vi "Plasma etching vacuum chamber automatization.vi"() -> ()   [LabVIEW 2019]
uses:
  <vilib>/MakerHub/LINX/Private/Type Defs/User Platform.ctl
  <vilib>/MakerHub/LINX/Public/Peripherals/Digital/Digital Read N Chans.vi
  <vilib>/MakerHub/LINX/Public/Peripherals/Digital/Digital Write N Chans.vi
  <vilib>/MakerHub/LINX/Public/Peripherals/Analog/Analog Read N Chans.vi
  <vilib>/MakerHub/LINX/Private/Local IO/LinxDigitalRead.vi
  <vilib>/MakerHub/LINX/Public/Utilities/Check Channel.vi
  <vilib>/MakerHub/LINX/Private/Local IO/LinxDigitalWrite.vi
  <vilib>/MakerHub/LINX/Private/Local IO/LinxAnalogRead.vi
  <vilib>/MakerHub/LINX/Private/Utilties/Generate Error.vi
  <vilib>/MakerHub/LINX/LMH-LINX.lvlib
panel:
  out "DIFFUSION PUMP HEATER VAR":bool
  in  "Tab Control":T1(tab)
  out "Back Air Admit":bool
  out "Chamber Valve":bool
  out "DIFF Valve":bool
  out "DIFFUSION PUMP Heater":bool
  out "Diafragma":bool
  out "Woter Exist":bool
  in  "Cold Woter Chamber":bool
  in  "Hot Woter  Chamber":bool
  out "Chamber Air Admit":bool
  out "Diff Pump Hot":bool
  out "Mechanic Pump":bool
  in  "Chamber Air Admit 2":bool
  out "Down Space Low Vacuum":dbl(knob) scale=0.0..1.0 scale format="%#_2g"
  in  "Chamber Open":bool
  in  "Chamber Close":bool
  out "Self Pumping":bool
  in  "Auto Start":bool
  in  "END Process":bool
  in  "STOP":bool
  out "Process Succesful ENDED":bool
  out "Vacuum Good":bool
  out "Chamber Low Vacuum":dbl(knob) scale=0.0..1.0 scale format="%#_2g"
  in  "Manual/Auto":bool
  out "Vacuum Measure":dbl(graph)
  out "High Vacuum Pascal":dbl format="%#_2e"
  in  "Serial Port":refnum<visa-resource-name>="COM12"
  in  "Diafragma Manual":bool
  in  "air Admit Manual":bool
  in  "Diff Pump Manual":bool
  in  "Chamber air Admit Manual":bool
  in  "DIFF VALVE Manual":bool
  in  "Mechanical Pump Manual":bool
  in  "CHAMBER VALVE Manual":bool
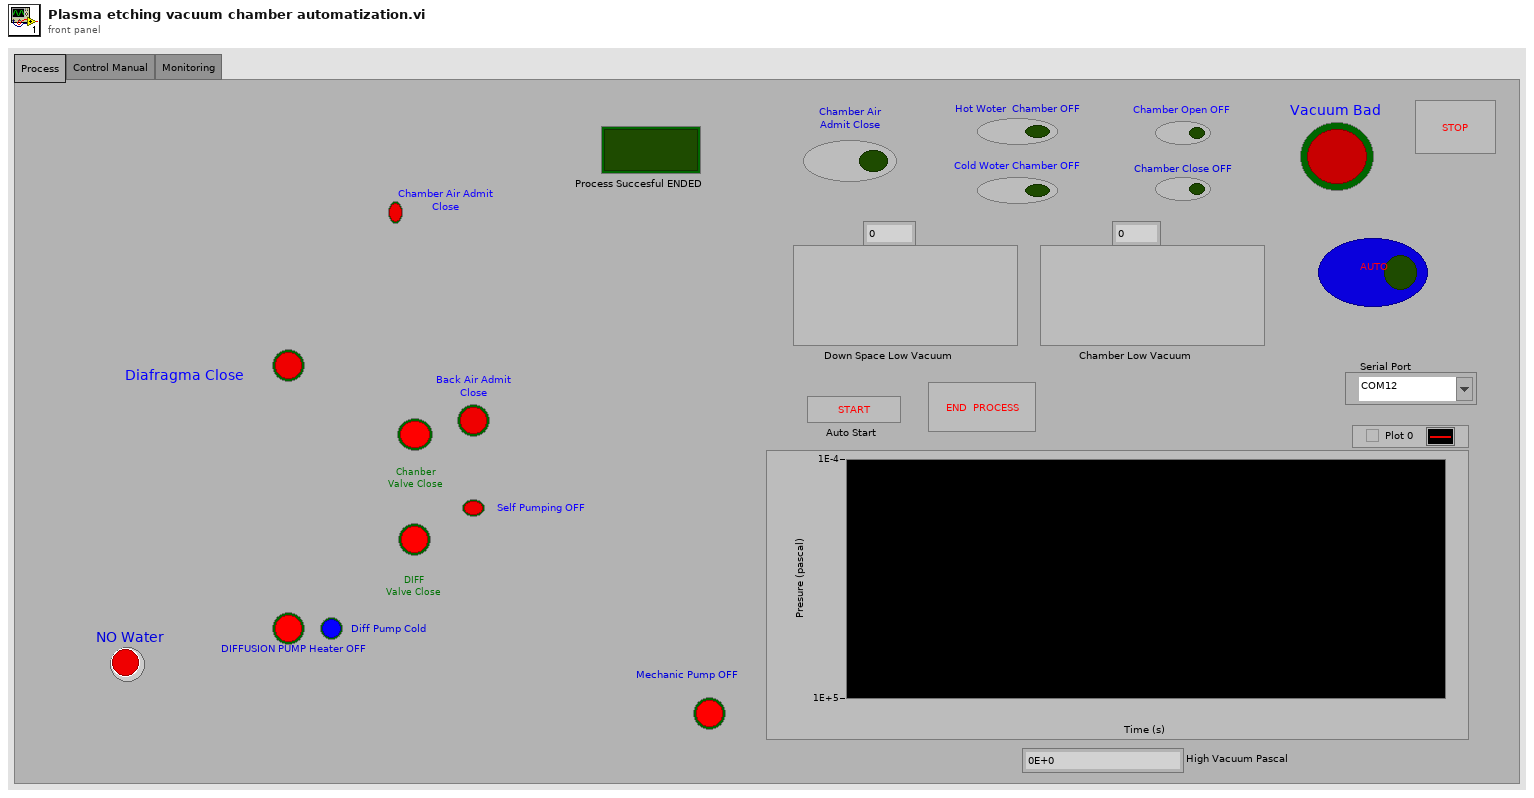
[diagram p1: front panel]
types:
  T1 = enum32{"Process", "Control Manual", "Monitoring"}
  T2 = typedef "LMH-LINX.lvlib/User Platform.ctl" = enum16{"Default", "Remote", "Local"}
  T3 = typedef "LMH-LINX.lvlib/LINX Ref.ctl" = cluster{"IO":T4, "Interface":T5, "LINX Device Config":T6}
  T4 = typedef "LMH-LINX.lvlib/Platform.ctl" = enum16{"Remote", "Local"}
  T5 = typedef "LMH-LINX.lvlib/Interface.ctl" = enum16{"Serial", "TCP"}
  T6 = typedef "LMH-LINX.lvlib/Device.lvlib/LINX Device Config.ctl" = cluster{"Interface":T5, "COM Port":refnum<visa-resource-name>, "TCP Configuration":T7, "Device Family":u8, "Device ID":u8, "Device Name":string, "TCP Ref":refnum<k5>, "Channels":T8}
  T7 = typedef "LMH-LINX.lvlib/Device.lvlib/TCP Config.ctl" = cluster{"IP Address":string, "Port":u16}
  T8 = typedef "LMH-LINX.lvlib/Channels.ctl" = cluster{"DI":u8[], "DO":u8[], "AI":u8[], "AO":u8[], "PWM":u8[], "QE":u8[], "UART":u8[], "I2C 2":u8[], "SPI":u8[], "CAN":u8[], "Servo":u8[], "AI Ref (V)":dbl, "AI Resolution (Bits)":u8, "AO Ref (V)":dbl, "AO Resolution (Bits)":u8}
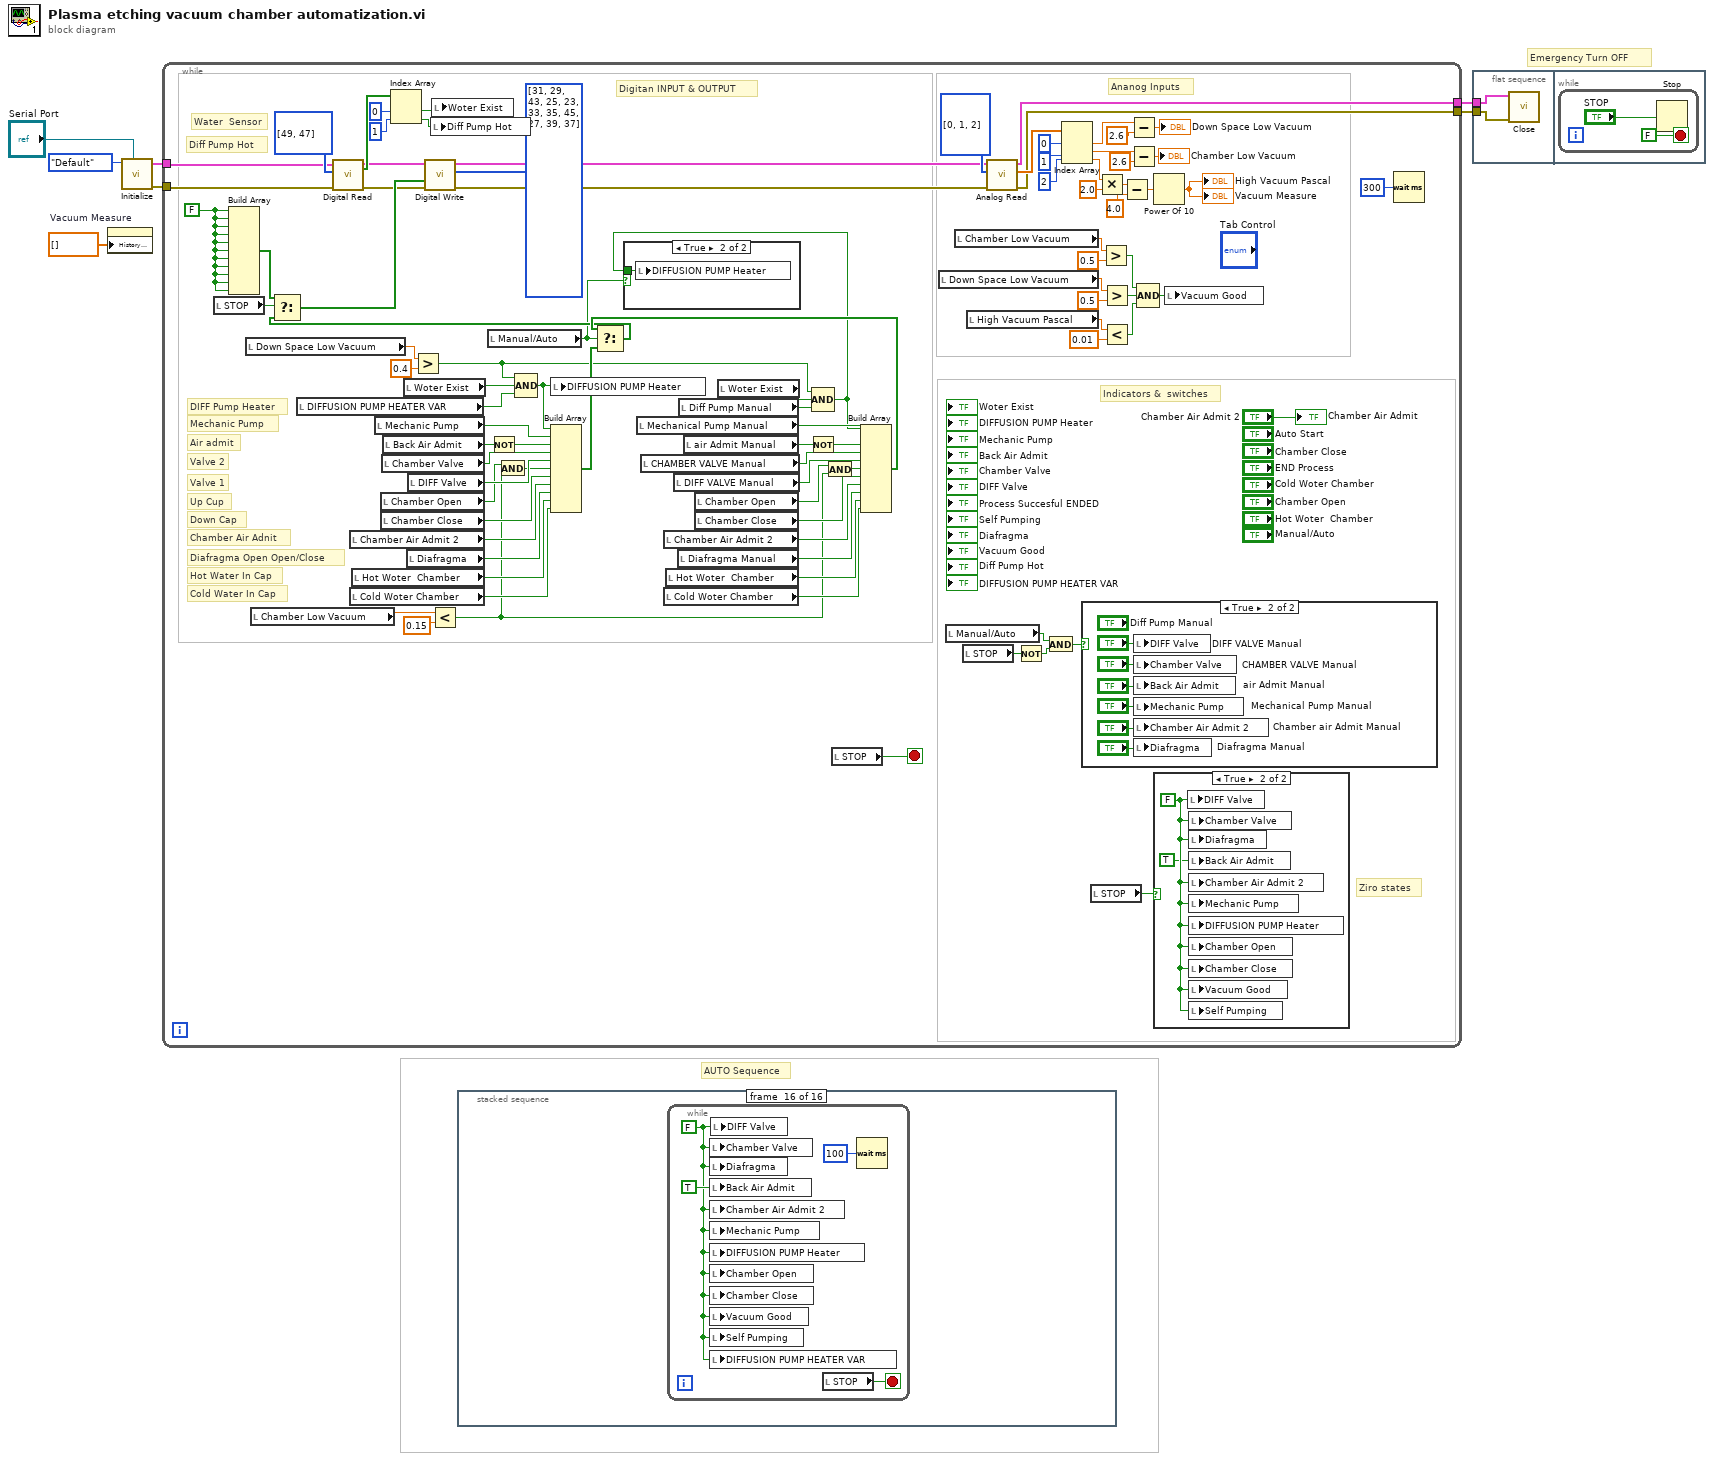
[diagram p0: block diagram]
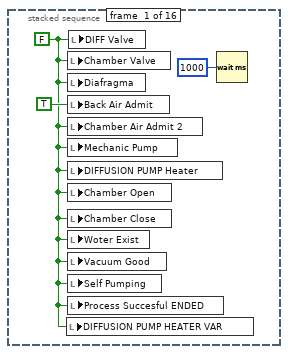
[diagram p2: hidden frame]
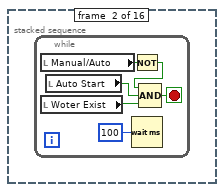
[diagram p3: hidden frame]
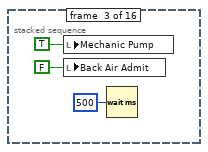
[diagram p4: hidden frame]
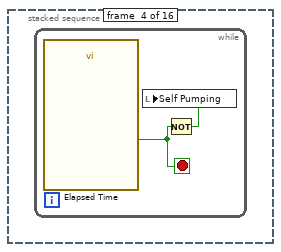
[diagram p5: hidden frame]
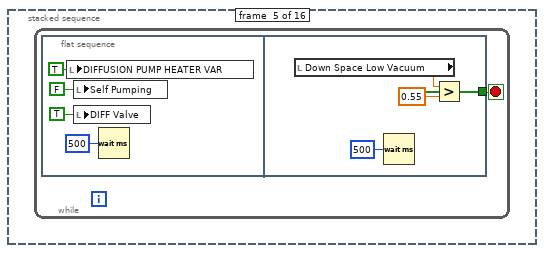
[diagram p6: hidden frame]
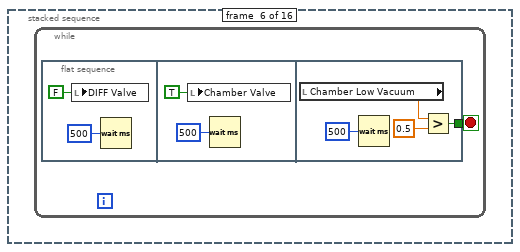
[diagram p7: hidden frame]
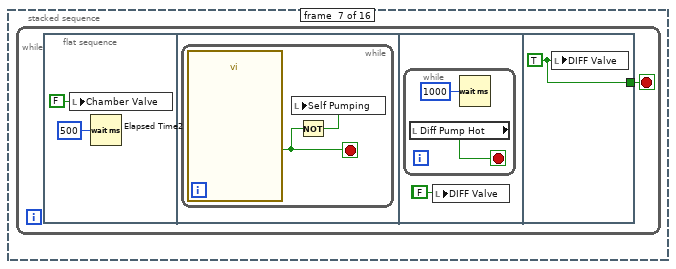
[diagram p8: hidden frame]
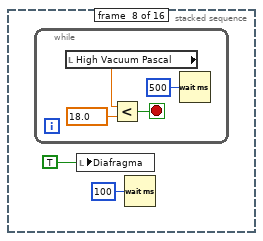
[diagram p9: hidden frame]
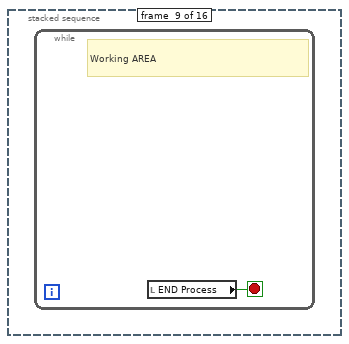
[diagram p10: hidden frame]
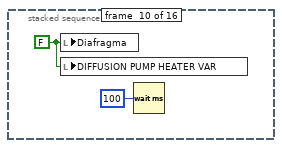
[diagram p11: hidden frame]
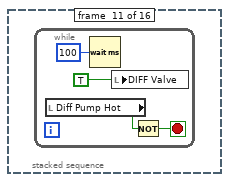
[diagram p12: hidden frame]
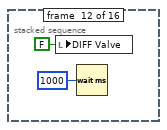
[diagram p13: hidden frame]
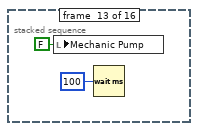
[diagram p14: hidden frame]
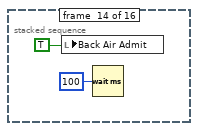
[diagram p15: hidden frame]
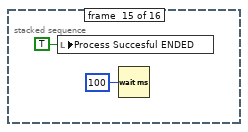
[diagram p16: hidden frame]
diagram:
  # "Emergency Turn OFF"
  # "AUTO Sequence"
  n1 = property on="Vacuum Measure" class="WFChart (strict)"("History Data"=dbl[] []) -> ()  [unwired: 2 in, 2 out]
  n2 = call <vilib>:"Initialize.vi"("Serial Port"="Serial Port", "IO"=User_Platform."Default" ("Platform")) -> ("Error Out"=w4:errorcluster, "LINX Resource"=w5:T3)  [unwired: 7 in, 1 out]
  n3 = while {
    tunnel: w5 -> [w52]
    tunnel: w4 -> [w51]
    tunnel: [w11] -> w3
    tunnel: [w10] -> w2
    stop <- w9 stop-if-true
    w58 = FALSE ("element")
    # "Ziro states"
    # "Indicators &  switches"
    # "Ananog Inputs"
    # "Diff Pump Hot"
    # "Cold Water In Cap"
    # "Hot Water In Cap"
    # "Diafragma Open Open/Close"
    # "Chamber Air Adnit"
    # "Down Cap"
    # "Up Cup"
    # "DIFF Pump Heater"
    # "Mechanic Pump"
    # "Air admit"
    # "Valve 2"
    # "Valve 1"
    # "Water  Sensor"
    # "Digitan INPUT & OUTPUT"
    n4 = local read "STOP"() -> (w54:bool)
    n5 = Build Array(w58, w58, w58, w58, w58, w58, w58, w58, w58, w58, w58) -> (w57:bool[])
    n6 = local read "Down Space Low Vacuum"() -> (w78:dbl)
    n7 = local read "Chamber Low Vacuum"() -> (w81:dbl)
    n8 = local read "DIFFUSION PUMP HEATER VAR"() -> (w59:bool)
    n9 = call-poly <vilib>:"Digital Read.vi"("Error In"=w51, "DI Channels"=u8[] [49, 47], "LINX Resource"=w52) -> ("Error Out"=w21:errorcluster, "Values"=w100:bool[], "LINX Resource"=w22:T3)  [unwired: 6 in]
    n10 = local read "Chamber Air Admit 2"() -> (w91:bool)
    n11 = local read "Cold Woter Chamber"() -> (w86:bool)
    n12 = local read "Hot Woter  Chamber"() -> (w87:bool)
    n13 = local read "Mechanic Pump"() -> (w98:bool)
    n14 = local read "Chamber Open"() -> (w82:bool)
    n15 = local read "Chamber Close"() -> (w92:bool)
    n16 = local read "Chamber Valve"() -> (w96:bool)
    n17 = local read "Back Air Admit"() -> (w84:bool)
    n18 = Index Array(array=w100, index #1=0 ("index"), index #2=1 ("index")) -> (element #1=w101:bool, element #2=w88:bool)
    n19 = local read "Woter Exist"() -> (w79:bool)
    n20 = local read "Diafragma"() -> (w90:bool)
    n21 = local read "DIFF Valve"() -> (w97:bool)
    n22 = Greater?(x=w78, y=0.4) -> (0:w63:bool)
    n23 = Less?(x=w81, y=0.15) -> (x < y?=w62:bool)
    n24 = local write "Diff Pump Hot"(w88) -> ()
    n25 = local write "Woter Exist"(w101) -> ()
    n26 = local read "Manual/Auto"() -> (w48:bool)
    n27 = Not(x=w84) -> (.not. x?=w85:bool)
    n28 = And(x=w82, y=w62) -> (x .and. y?=w83:bool)
    n29 = Compound Arithmetic op=AND(w63, w79, w59) -> (w60:bool)
    n30 = local write "DIFFUSION PUMP Heater"(w60) -> ()
    n31 = Build Array(w60, w98, w85, w96, w97, w83, w92, w91, w90, w87, w86) -> (w64:bool[])
    n32 = local read "Mechanical Pump Manual"() -> (w67:bool)
    n33 = local read "CHAMBER VALVE Manual"() -> (w66:bool)
    n34 = local read "Chamber Air Admit 2"() -> (w72:bool)
    n35 = local read "Cold Woter Chamber"() -> (w75:bool)
    n36 = local read "Hot Woter  Chamber"() -> (w74:bool)
    n37 = local read "DIFF VALVE Manual"() -> (w65:bool)
    n38 = local read "Diafragma Manual"() -> (w73:bool)
    n39 = local read "Diff Pump Manual"() -> (w49:bool)
    n40 = local read "air Admit Manual"() -> (w70:bool)
    n41 = local read "Chamber Open"() -> (w50:bool)
    n42 = local read "Chamber Close"() -> (w71:bool)
    n43 = local read "Woter Exist"() -> (w68:bool)
    n44 = Not(x=w70) -> (.not. x?=w69:bool)
    n45 = Compound Arithmetic op=AND(w63, w68, w49) -> (w53:bool)
    n46 = case shown="True" w48 {
      tunnel: w53 -> [_ w110]
      frame False {
      }
      frame True {
        n47 = local write "DIFFUSION PUMP Heater"(w110) -> ()
      }
    }
    n48 = And(x=w50, y=w62) -> (x .and. y?=w61:bool)
    n49 = local read "STOP"() -> (w9:bool)
    n50 = Build Array(w53, w67, w69, w66, w65, w61, w71, w72, w73, w74, w75) -> (w76:bool[])
    n51 = Select(t=w76, s=w48, f=w64) -> (s? t:f=w55:bool[])
    n52 = Select(t=w57, s=w54, f=w55) -> (s? t:f=w56:bool[])
    n53 = call-poly <vilib>:"Digital Write.vi"("Error In"=w21, "Values"=w56, "DO Channels"=u8[] [31, 29, 43, 25, 23, 33, 35, 45, 27, 39, 37], "LINX Resource"=w22) -> ("Error Out"=w19:errorcluster, "LINX Resource"=w20:T3)  [unwired: 6 in]
    n54 = local read "Down Space Low Vacuum"() -> (w33:dbl)
    n55 = local read "Manual/Auto"() -> (w14:bool)
    n56 = local read "Chamber Low Vacuum"() -> (w36:dbl)
    n57 = local read "STOP"() -> (w13:bool)
    n58 = local read "High Vacuum Pascal"() -> (w32:dbl)
    n59 = call-poly <vilib>:"Analog Read.vi"("Error In"=w19, "AI Channel(s)"=u8[] [0, 1, 2], "LINX Resource"=w20) -> ("Error Out"=w10:errorcluster, "Voltages"=w27:dbl[], "LINX Resource"=w11:T3)  [unwired: 5 in, 1 out]
    n60 = Not(x=w13) -> (.not. x?=w12:bool)
    n61 = And(x=w14, y=w12) -> (x .and. y?=w15:bool)
    n62 = Index Array(array=w27, index #1=0 ("index"), index #2=1 ("index"), index #3=2 ("index")) -> (element #1=w28:dbl, element #2=w41:dbl, element #3=w18:dbl)
    n63 = case shown="True" w15 {
      frame False {
      }
      frame True {
        n64 = local write "DIFF Valve"("DIFF VALVE Manual") -> ()
        n65 = local write "Chamber Valve"("CHAMBER VALVE Manual") -> ()
        n66 = local write "Back Air Admit"("air Admit Manual") -> ()
        n67 = local write "Mechanic Pump"("Mechanical Pump Manual") -> ()
        n68 = local write "Chamber Air Admit 2"("Chamber air Admit Manual") -> ()
        n69 = local write "Diafragma"("Diafragma Manual") -> ()
      }
    }
    n70 = local read "STOP"() -> (w8:bool)
    n71 = Multiply(x=w18, y=2.0 ("x")) -> (x*y=w47:dbl)
    n72 = Greater?(x=w36, y=0.5) -> (0:w37:bool)
    n73 = Greater?(x=w33, y=0.5) -> (0:w38:bool)
    n74 = Less?(x=w32, y=0.01) -> (x < y?=w39:bool)
    n75 = Subtract(x=w47, y=4.0) -> (x-y=w45:dbl)
    n76 = Subtract(x=w28, y=2.6) -> (x-y=→"Down Space Low Vacuum":dbl)
    n77 = Subtract(x=w41, y=2.6) -> (x-y=→"Chamber Low Vacuum":dbl)
    n78 = Compound Arithmetic op=AND(w37, w38, w39) -> (w40:bool)
    n79 = Power Of 10(x=w45) -> (10^x=→"High Vacuum Pascal" →"Vacuum Measure":dbl)
    n80 = case shown="True" w8 {
      frame False {
      }
      frame True {
        w103 = FALSE ("Process Sucesfull ENDED")
        n81 = local write "DIFF Valve"(w103) -> ()
        n82 = local write "Chamber Valve"(w103) -> ()
        n83 = local write "Diafragma"(w103) -> ()
        n84 = local write "Back Air Admit"(TRUE ("Back Air Admit")) -> ()
        n85 = local write "Chamber Air Admit 2"(w103) -> ()
        n86 = local write "Mechanic Pump"(w103) -> ()
        n87 = local write "DIFFUSION PUMP Heater"(w103) -> ()
        n88 = local write "Chamber Open"(w103) -> ()
        n89 = local write "Chamber Close"(w103) -> ()
        n90 = local write "Vacuum Good"(w103) -> ()
        n91 = local write "Self Pumping"(w103) -> ()
      }
    }
    n92 = local write "Vacuum Good"(w40) -> ()
    n93 = Wait (ms)(milliseconds to wait=u32 300) -> ()  [unwired: 1 out]
    "Chamber Air Admit" <- "Chamber Air Admit 2"
  }
  n94 = stacked-sequence {
    frame #0 {
      w111 = FALSE ("Process Sucesfull ENDED")
      n95 = local write "DIFFUSION PUMP HEATER VAR"(w111) -> ()
      n96 = local write "Chamber Valve"(w111) -> ()
      n97 = local write "Diafragma"(w111) -> ()
      n98 = local write "Back Air Admit"(TRUE ("Back Air Admit")) -> ()
      n99 = local write "Chamber Air Admit 2"(w111) -> ()
      n100 = local write "Mechanic Pump"(w111) -> ()
      n101 = local write "DIFFUSION PUMP Heater"(w111) -> ()
      n102 = local write "Chamber Open"(w111) -> ()
      n103 = local write "Chamber Close"(w111) -> ()
      n104 = local write "Woter Exist"(w111) -> ()
      n105 = local write "Vacuum Good"(w111) -> ()
      n106 = local write "Self Pumping"(w111) -> ()
      n107 = local write "Process Succesful ENDED"(w111) -> ()
      n108 = local write "DIFF Valve"(w111) -> ()
      n109 = Wait (ms)(milliseconds to wait=u32 1000) -> ()  [unwired: 1 out]
    }
    frame #1 {
      n110 = while {
        stop <- w114 stop-if-true
        n111 = local read "Manual/Auto"() -> (w118:bool)
        n112 = local read "Woter Exist"() -> (w117:bool)
        n113 = local read "Auto Start"() -> (w115:bool)
        n114 = Not(x=w118) -> (.not. x?=w116:bool)
        n115 = Wait (ms)(milliseconds to wait=u32 100) -> ()  [unwired: 1 out]
        n116 = Compound Arithmetic op=AND(w116, w115, w117) -> (w114:bool)
      }
    }
    frame #2 {
      n117 = local write "Mechanic Pump"(TRUE ("Mechanic Pump")) -> ()
      n118 = local write "Back Air Admit"(FALSE ("Back Air Admit")) -> ()
      n119 = Wait (ms)(milliseconds to wait=u32 500) -> ()  [unwired: 1 out]
    }
    frame #3 {
      n120 = while {
        stop <- w123 stop-if-true
        n121 = call "Elapsed Time"() -> ("Time has Elapsed"=w123:bool)  [unwired: 12 in, 7 out]
        n122 = Not(x=w123) -> (.not. x?=w124:bool)
        n123 = local write "Self Pumping"(w124) -> ()
      }
    }
    frame #4 {
      n124 = while {
        stop <- w125 stop-if-true
        n125 = flat-sequence {
          tunnel: [w130] -> w125
          frame #0 {
            n126 = local write "DIFFUSION PUMP HEATER VAR"(TRUE ("DIFFUSION PUMP HEATER VAR")) -> ()
            n127 = local write "Self Pumping"(FALSE ("Self Pumping")) -> ()
            n128 = local write "DIFF Valve"(TRUE ("valve 1")) -> ()
            n129 = Wait (ms)(milliseconds to wait=u32 500) -> ()  [unwired: 1 out]
          }
          frame #1 {
            n130 = local read "Down Space Low Vacuum"() -> (w133:dbl)
            n131 = Wait (ms)(milliseconds to wait=u32 500) -> ()  [unwired: 1 out]
            n132 = Greater?(x=w133, y=0.55) -> (0:w130:bool)
          }
        }
      }
    }
    frame #5 {
      n133 = while {
        stop <- w134 stop-if-true
        n134 = flat-sequence {
          tunnel: [w140] -> w134
          frame #0 {
            n135 = local write "DIFF Valve"(FALSE ("valve 1")) -> ()
            n136 = Wait (ms)(milliseconds to wait=u32 500) -> ()  [unwired: 1 out]
          }
          frame #1 {
            n137 = local write "Chamber Valve"(TRUE ("valve 2")) -> ()
            n138 = Wait (ms)(milliseconds to wait=u32 500) -> ()  [unwired: 1 out]
          }
          frame #2 {
            n139 = local read "Chamber Low Vacuum"() -> (w141:dbl)
            n140 = Wait (ms)(milliseconds to wait=u32 500) -> ()  [unwired: 1 out]
            n141 = Greater?(x=w141, y=0.5) -> (0:w140:bool)
          }
        }
      }
    }
    frame #6 {
      n142 = while {
        stop <- w143 stop-if-true
        n143 = flat-sequence {
          tunnel: [w151] -> w143
          frame #0 {
            n144 = local write "Chamber Valve"(FALSE ("valve 2")) -> ()
            n145 = Wait (ms)(milliseconds to wait=u32 500) -> ()  [unwired: 1 out]
          }
          frame #1 {
            n146 = while {
              stop <- w146 stop-if-true
              n147 = call "Elapsed Time2"() -> ("Time has Elapsed"=w146:bool)  [unwired: 12 in, 7 out]
              n148 = Not(x=w146) -> (.not. x?=w147:bool)
              n149 = local write "Self Pumping"(w147) -> ()
            }
          }
          frame #2 {
            (unwired) FALSE ("valve 2")
            n150 = while {
              stop <- w149 stop-if-true
              n151 = local read "Diff Pump Hot"() -> (w149:bool)
              n152 = Wait (ms)(milliseconds to wait=u32 1000) -> ()  [unwired: 1 out]
            }
            n153 = local write "DIFF Valve"(TRUE ("valve 2")) -> ()
          }
          frame #3 {
            w151 = TRUE ("valve 1")
            n154 = local write "DIFF Valve"(w151) -> ()
          }
        }
      }
    }
    frame #7 {
      n155 = while {
        stop <- w155 stop-if-true
        n156 = local read "High Vacuum Pascal"() -> (w157:dbl)
        n157 = Less?(x=w157, y=18.0) -> (x < y?=w155:bool)
        n158 = Wait (ms)(milliseconds to wait=u32 500) -> ()  [unwired: 1 out]
      }
      n159 = local write "Diafragma"(TRUE ("Diafragma Open")) -> ()
      n160 = Wait (ms)(milliseconds to wait=u32 100) -> ()  [unwired: 1 out]
    }
    frame #8 {
      n161 = while {
        stop <- w158 stop-if-true
        # "Working AREA"
        n162 = local read "END Process"() -> (w158:bool)
      }
    }
    frame #9 {
      w160 = FALSE
      n163 = local write "Diafragma"(w160) -> ()
      n164 = local write "DIFFUSION PUMP HEATER VAR"(w160) -> ()
      n165 = Wait (ms)(milliseconds to wait=u32 100) -> ()  [unwired: 1 out]
    }
    frame #10 {
      n166 = while {
        stop <- w163 stop-if-true
        n167 = local read "Diff Pump Hot"() -> (w162:bool)
        n168 = Wait (ms)(milliseconds to wait=u32 100) -> ()  [unwired: 1 out]
        n169 = local write "DIFF Valve"(TRUE) -> ()
        n170 = Not(x=w162) -> (.not. x?=w163:bool)
      }
    }
    frame #11 {
      n171 = local write "DIFF Valve"(FALSE ("valve 1")) -> ()
      n172 = Wait (ms)(milliseconds to wait=u32 1000) -> ()  [unwired: 1 out]
    }
    frame #12 {
      n173 = local write "Mechanic Pump"(FALSE ("Mechanic Pump")) -> ()
      n174 = Wait (ms)(milliseconds to wait=u32 100) -> ()  [unwired: 1 out]
    }
    frame #13 {
      n175 = local write "Back Air Admit"(TRUE) -> ()
      n176 = Wait (ms)(milliseconds to wait=u32 100) -> ()  [unwired: 1 out]
    }
    frame #14 {
      n177 = local write "Process Succesful ENDED"(TRUE ("Process Sucesfull ENDED")) -> ()
      n178 = Wait (ms)(milliseconds to wait=u32 100) -> ()  [unwired: 1 out]
    }
    frame #15 {
      n179 = while {
        stop <- w175 stop-if-true
        w173 = FALSE ("Process Sucesfull ENDED")
        n180 = local write "Chamber Valve"(w173) -> ()
        n181 = local write "Diafragma"(w173) -> ()
        n182 = local write "Back Air Admit"(TRUE ("Back Air Admit")) -> ()
        n183 = local write "Chamber Air Admit 2"(w173) -> ()
        n184 = local write "Mechanic Pump"(w173) -> ()
        n185 = local write "DIFFUSION PUMP Heater"(w173) -> ()
        n186 = local write "Chamber Open"(w173) -> ()
        n187 = local write "Chamber Close"(w173) -> ()
        n188 = local write "Vacuum Good"(w173) -> ()
        n189 = local write "Self Pumping"(w173) -> ()
        n190 = local write "DIFFUSION PUMP HEATER VAR"(w173) -> ()
        n191 = local write "DIFF Valve"(w173) -> ()
        n192 = local read "STOP"() -> (w175:bool)
        n193 = Wait (ms)(milliseconds to wait=u32 100) -> ()  [unwired: 1 out]
      }
    }
  }
  n194 = flat-sequence {
    tunnel: w2 -> [w178]
    tunnel: w3 -> [w177]
    frame #0 {
      n195 = call <vilib>:"Close.vi"("Error In"=w178, "LINX Resource"=w177) -> ()  [unwired: 9 in, 1 out]
    }
    frame #1 {
      n196 = while {
        stop <- FALSE stop-if-true
        n197 = Stop(stop? (T)="STOP") -> ()
      }
    }
  }
